vi "AddressN1911A.vi"() -> (0 "Port":i32=5025 min=0 max=65535 step=1 format="%_5g", 1 "IP address":string)   [LabVIEW 2009]
doc: "Provdes the IP address and TCP/IP port number\nfor the N1911A power meter"
panel:
  in  "IP address":string="10.1.10.101"
  in  "Port":i32=5025 min=0 max=65535 step=1 format="%_5g"
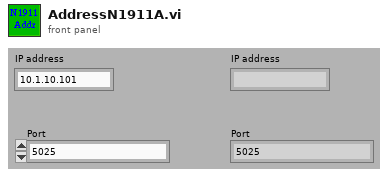
[diagram p1: front panel]
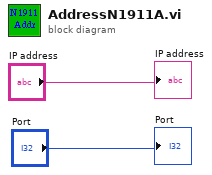
[diagram p0: block diagram]
diagram:
  "Port" <- "Port"
  "IP address" <- "IP address"
